vi "InverseMpemba_HotColdWarm_test.vi"(6 "RN":sgl, 8 "X0":sgl=0.5, 11 "array":sgl[](array[numeric])) -> (3 "Xpot":sgl, 5 "dx":sgl)   [LabVIEW 2019]
uses:
  <vilib>/Platform/TimedLoop/XDataNode/timing_clust.ctl
  <vilib>/Platform/TimedLoop/XDataNode/nitl_modes.ctl
  <vilib>/Platform/TimedLoop/XDataNode/wakeup.ctl
  <vilib>/Platform/TimedLoop/XDataNode/XDataNode.xnode
  <vilib>/Platform/TimedLoop/XDataNode/XDNodeRunTimeDep.lvlib
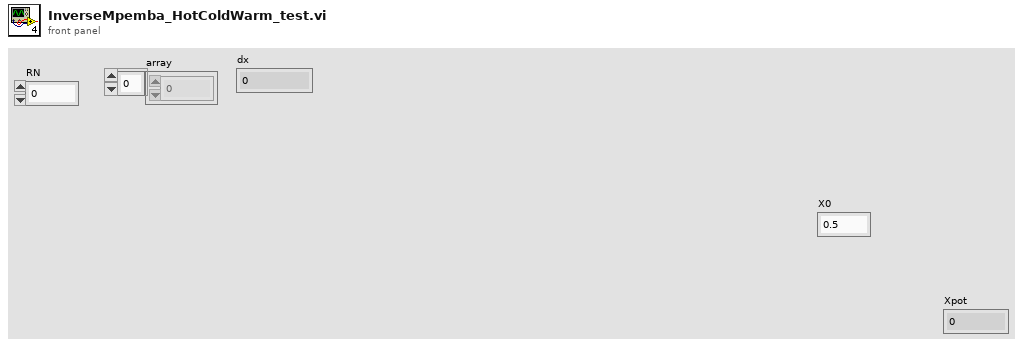
[diagram p1: front panel]
types:
  T1 = typedef "XDNodeRunTimeDep.lvlib/timing_clust.ctl" = cluster{"Expected End [f-1]":u64, "Actual End [f-1]":u64, "Finished Late? [f-1]":bool, "Expected End [i-1]":u64, "Actual End [i-1]":u64, "Finished Late? [i-1]":bool, "Expected Start [i]":u64, "Actual Start [i]":u64, "Expected Start [f]":u64, "Actual Start [f]":u64, "Source Name":string, "Structure Name":string, "Period":i64, "Deadline":i64, "Offset":i64, "Start":i64, "Priority":i32, "Timeout":i32, "Mode":T2, "Wakeup Reason":T3, "Error":errorcluster, "Source Type":string, "Secondary Source Type":string, "Global End Time":u64, "Global Start Time":u64, "Frame Duration":u64, "Iteration Duration":u64, "Assigned CPU":i32, "I/O Scan Engine Mode":u32}
  T2 = typedef "XDNodeRunTimeDep.lvlib/nitl_modes.ctl" = enum32{"No Change", "Process missed periods, maintain original phase", "Discard missed periods, maintain original phase", "Process missed periods, ignore original phase", "Discard missed periods, ignore original phase"}
  T3 = typedef "XDNodeRunTimeDep.lvlib/wakeup.ctl" = enum32{"Normal", "Aborted", "Asynchronous wakeup", "Timing source error", "Timed loop error", "Timeout"}
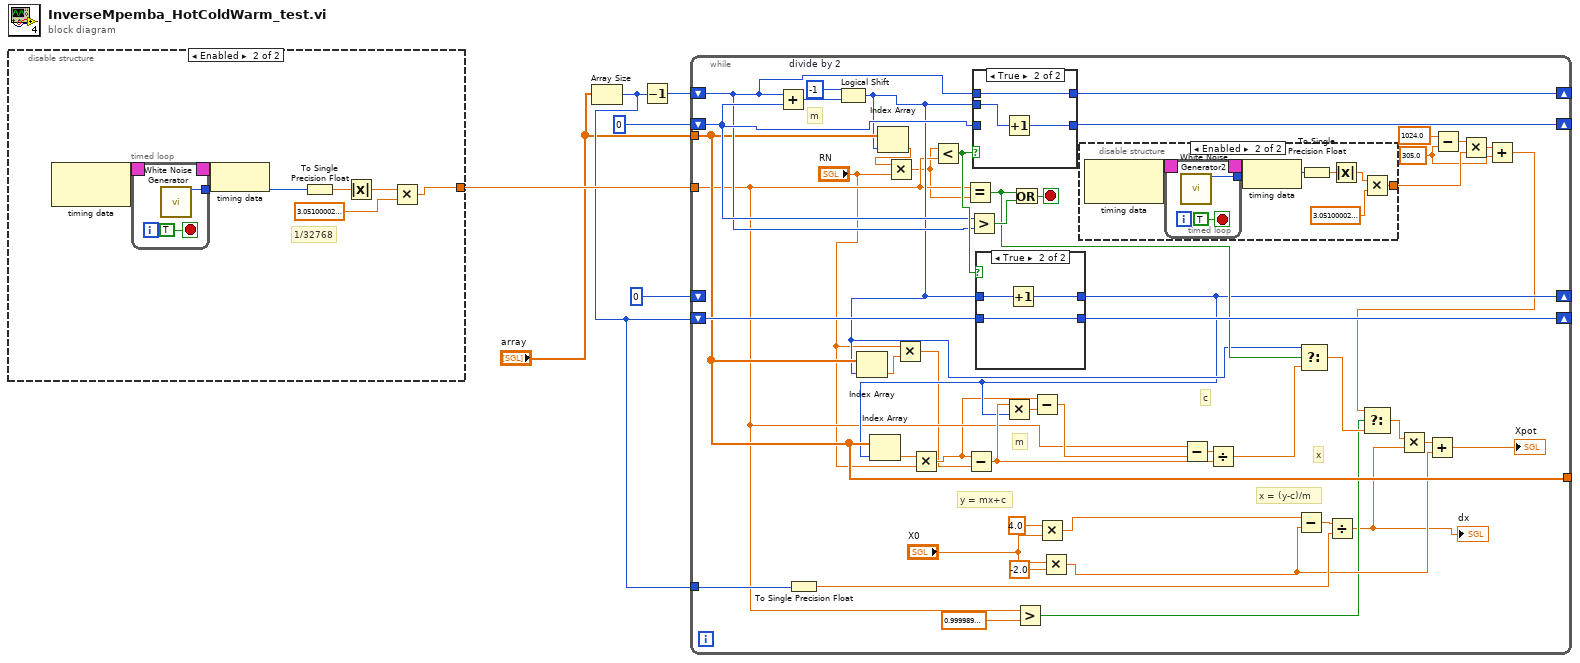
[diagram p0: block diagram]
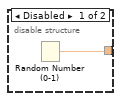
[diagram p2: hidden frame]
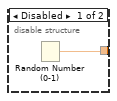
[diagram p3: hidden frame]
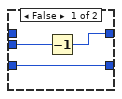
[diagram p5: hidden frame]
diagram:
  n1 = disable-structure shown="Enabled" {
    disable-tunnel: [w7 w10] -> w3
    frame Disabled {
      n2 = Random Number (0-1)() -> (number: 0 to 1=w7:dbl)
    }
    frame Enabled {
      # "1/32768"
      n3 = node-c288() -> (w9:T1)  [unwired: 1 in]
      n4 = timed-loop {
        timing: w9 -> [_]
        timing-out: [_] -> w8
        tunnel: [w16] -> w14
        stop <- TRUE stop-if-true
        n5 = call "White Noise Generator"() -> ("white noise out"=w16:i16)  [unwired: 15 in]
      }
      n6 = node-c288(w8) -> ()
      n7 = To Single Precision Float(number=w14) -> (single precision float=w12:sgl)
      n8 = Absolute Value(x=w12) -> (abs(x)=w11:sgl)
      n9 = Multiply(x=w11, y=sgl 3.051e-05) -> (x*y=w10:sgl)
    }
  }
  n10 = Array Size(array="array") -> (size(s)=w2:i32)
  n11 = Decrement(x=w2) -> (x-1=w4:i32)
  n12 = while {
    tunnel: "array" -> [w58]
    tunnel: w3 -> [w40]
    shift-right: [w68] -> _
    shift-left: w4 -> [w59]
    shift-right: [w64] -> _
    shift-left: 0 -> [w60]
    shift-right: [w50] -> _
    shift-left: 0 -> [_]
    shift-right: [w61] -> _
    shift-left: w2 -> [w62]
    tunnel: [w58] -> _
    tunnel: w2 -> [w45]
    stop <- w66 stop-if-true
    w33 = sgl 305.0 ("y")
    w69 = -1  # divide by 2
    # "x"
    # "x = (y-c)/m"
    # "c"
    # "m"
    # "y = mx+c"
    # "m"
    n13 = Add(x=w59, y=w60) -> (x+y=w65:i32)
    n14 = To Single Precision Float(number=w45) -> (single precision float=w44:sgl)
    n15 = Logical Shift(y=w69, x=w65) -> (x << y=w56:i32)
    n16 = Index Array(array=w58, index=w56) -> (element=w25:sgl)
    n17 = Index Array(array=w58, index=w56) -> (element=w29:sgl)
    n18 = Multiply(x=w29, y="RN") -> (x*y=w28:sgl)
    n19 = Multiply(x="RN", y=w25) -> (x*y=w23:sgl)
    n20 = Less?(x=w28, y=w40) -> (x < y?=w63:bool)
    n21 = Equal?(x=w40, y=w28) -> (x = y?=w57:bool)
    n22 = Greater?(x=w60, y=w59) -> (0:w67:bool)
    n23 = case shown="True" w63 {
      tunnel: w56 -> [w91 w94]
      tunnel: [w90 w92] -> w68
      tunnel: w60 -> [w89 _]
      tunnel: [w89 w93] -> w64
      tunnel: w59 -> [_ w92]
      frame False {
        n24 = Decrement(x=w91) -> (x-1=w90:i32)
      }
      frame True {
        n25 = Increment(x=w94) -> (x+1=w93:i32)
      }
    }
    n26 = case shown="True" w63 {
      tunnel: w56 -> [w85 w88]
      tunnel: [w84 w87] -> w50
      tunnel: w62 -> [w84 w86]
      tunnel: [w85 w86] -> w61
      frame False {
      }
      frame True {
        n27 = Increment(x=w88) -> (x+1=w87:i32)
      }
    }
    n28 = Index Array(array=w58, index=w50) -> (element=w27:sgl)
    n29 = Multiply(x=w27, y="RN") -> (x*y=w26:sgl)
    n30 = Subtract(x=w26, y=w23) -> (x-y=w52:sgl)
    n31 = Multiply(x=w52, y=w50) -> (x*y=w55:sgl)
    n32 = Or(x=w57, y=w67) -> (x .or. y?=w66:bool)
    n33 = Greater?(x=w40, y=sgl 0.99999) -> (0:w30:bool)
    n34 = Subtract(x=w26, y=w55) -> (x-y=w54:sgl)
    n35 = Multiply(x=sgl 4.0, y="X0") -> (x*y=w47:sgl)
    n36 = Multiply(x="X0", y=sgl -2.0) -> (x*y=w42:sgl)
    n37 = disable-structure shown="Enabled" {
      disable-tunnel: [w70 w73] -> w35
      frame Disabled {
        n38 = Random Number (0-1)() -> (number: 0 to 1=w70:dbl)
      }
      frame Enabled {
        n39 = node-c288() -> (w72:T1)  [unwired: 1 in]
        n40 = timed-loop {
          timing: w72 -> [_]
          timing-out: [_] -> w71
          tunnel: [w79] -> w77
          stop <- TRUE stop-if-true
          n41 = call "White Noise Generator2"() -> ("white noise out"=w79:i16)  [unwired: 15 in]
        }
        n42 = node-c288(w71) -> ()
        n43 = To Single Precision Float(number=w77) -> (single precision float=w75:sgl)
        n44 = Absolute Value(x=w75) -> (abs(x)=w74:sgl)
        n45 = Multiply(x=w74, y=sgl 3.051e-05) -> (x*y=w73:sgl)
      }
    }
    n46 = Subtract(x=w40, y=w54) -> (x-y=w53:sgl)
    n47 = Divide(x=w53, y=w52) -> (x/y=w51:sgl)
    n48 = Subtract(x=w47, y=w42) -> (x-y=w46:sgl)
    n49 = Select(t=w56, s=w57, f=w51) -> (s? t:f=w38:sgl)
    n50 = Divide(x=w46, y=w44) -> (x/y=w21:sgl)
    "dx" <- w21
    n51 = Subtract(x=sgl 1024.0, y=w33) -> (x-y=w36:sgl)
    n52 = Multiply(x=w36, y=w35) -> (x*y=w34:sgl)
    n53 = Add(x=w34, y=w33) -> (x+y=w31:sgl)
    n54 = Select(t=w31, s=w30, f=w38) -> (s? t:f=w32:sgl)
    n55 = Multiply(x=w32, y=w21) -> (x*y=w43:sgl)
    n56 = Add(x=w43, y=w42) -> (x+y=→"Xpot":sgl)
  }
